vi "setAndorErrorCode.vi"(8 "error in (no error)":errorcluster, 10 "Andor Error Codes":dbl[](array[numeric]), 11 "AndorController.lvclass in":refnum<class "AndorController.lvclass">) -> (0 "error out":errorcluster, 3 "AndorController.lvclass out":refnum<class "AndorController.lvclass">)   [LabVIEW 2009, in "Hardware.lvlib" / "Channels.lvlib" / "AndorController.lvclass"]
uses:
  AndorController.lvclass
  AndorController.lvclass/AndorController.ctl
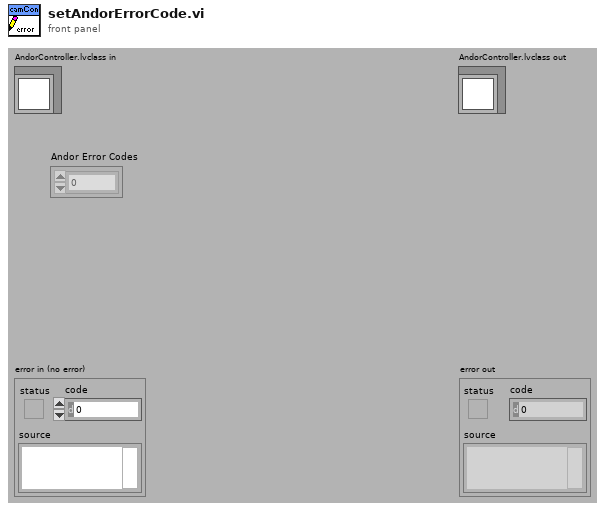
[diagram p1: front panel]
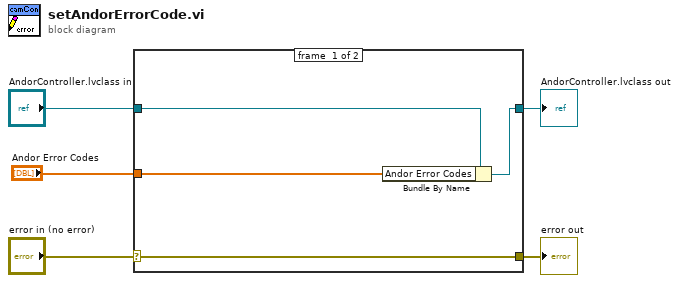
[diagram p0: block diagram]
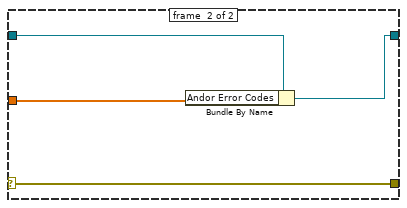
[diagram p2: hidden frame]
diagram:
  n1 = case shown="No Error" "error in (no error)" {
    selector: "error in (no error)" -> [w9 w11]
    tunnel: [w9 w11] -> w4
    tunnel: [w7 w12] -> w2
    tunnel: "AndorController.lvclass in" -> [w8 w13]
    tunnel: "Andor Error Codes" -> [w6 w10]
    frame #0 {
      n2 = Bundle By Name(cluster=w8, "Andor Error Codes"=w6) -> (w7:refnum<class "AndorController.lvclass">)
    }
    frame #1 {
      n3 = Bundle By Name(cluster=w13, "Andor Error Codes"=w10) -> (w12:refnum<class "AndorController.lvclass">)
    }
  }
  "error out" <- w4
  "AndorController.lvclass out" <- w2
